vi "Fetch(Y)Trace.vi"(8 "error in (no error)":errorcluster, 11 "Keysight44xx in":refnum<class "Keysight44xx.lvclass">) -> (0 "error out":errorcluster, 2 "Waveform(s)":T1, 3 "Keysight44xx out":refnum<class "Keysight44xx.lvclass">)   [LabVIEW 2018, in "SpecAnPlugins.lvlib" / "Keysight44xx.lvclass"]
doc: "This function returns the trace the spectrum analyzer acquires. The trace is from a previously initiated acquisition. The user calls the Initiate function to start an acquisition. The user calls the Acquisition Status function to determine when the acquisition is complete. \n\nThe user may call the Read Y Trace function instead of the Initiate function. This function starts an acquisition, waits for the acquisition to complete, and returns the trace in one function call. \n\nThe Amplitude array returns data that represents the amplitude of the signals obtained by sweeping from the start frequency to the stop frequency (in frequency domain, in the time domain the amplitude array is ordered from beginning of sweep to end). The Amplitude Units attribute determines the units of the points in the Amplitude array.\n\nThis function does not check the instrument status. The user calls the Error Query function at the conclusion of the sequence to check the instrument status."
uses:
  Keysight44xx.lvclass
  C:/Users/ico/Documents/Projects/NistPluggableModules/SpecAn/SpecAnPlugins/SpecAnBaseClass/SpecAnBase.lvclass
  SpecAnBaseClass/Typedefs/Waveform(s).ctl
  SpecAnBaseClass/SpecAnBase.lvclass
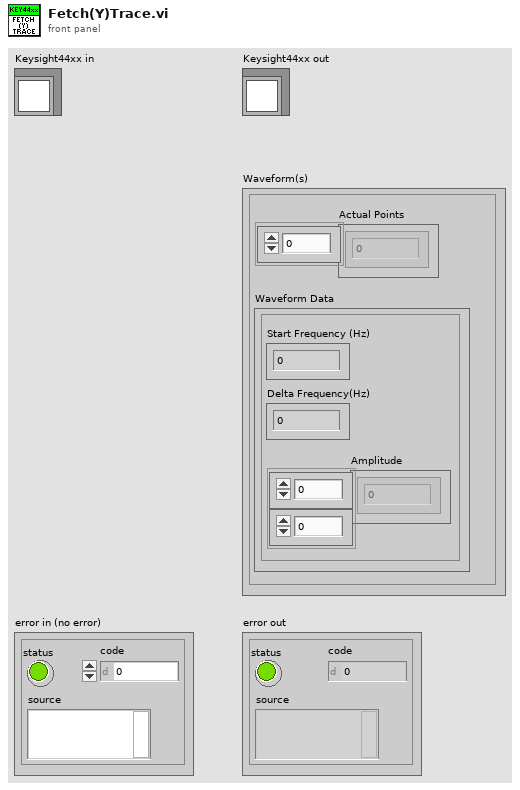
[diagram p1: front panel]
types:
  T1 = typedef "SpecAnPlugins.lvlib/SpecAnBase.lvclass/Waveform(s).ctl" = cluster{"Actual Points":i32[], "Waveform Data":cluster{"Start Frequency (Hz)":dbl, "Delta Frequency(Hz)":dbl, "Amplitude":dbl[][]}}
  T2 = typedef "SpecAnPlugins.lvlib/SpecAnBase.lvclass/Acquisition.ctl" = cluster{"Handle":string, "Connected":bool, "Enabled":bool, "SweepModeContinuous":bool, "NumberOfSweeps":i32, "DetectorTypeAuto":bool, "DetectorType":i32, "VerticalScale":i32, "MaximumTime(seconds)":dbl}
  T3 = typedef "SpecAnPlugins.lvlib/SpecAnBase.lvclass/Trace.ctl" = cluster{"TraceName":string, "TraceSize":i32, "TraceType":i32}[]
  T4 = typedef "SpecAnPlugins.lvlib/SpecAnBase.lvclass/Frequency.ctl" = cluster{"FrequencyStart":dbl, "FrequencyStop":dbl, "FrequencyOffset":dbl}
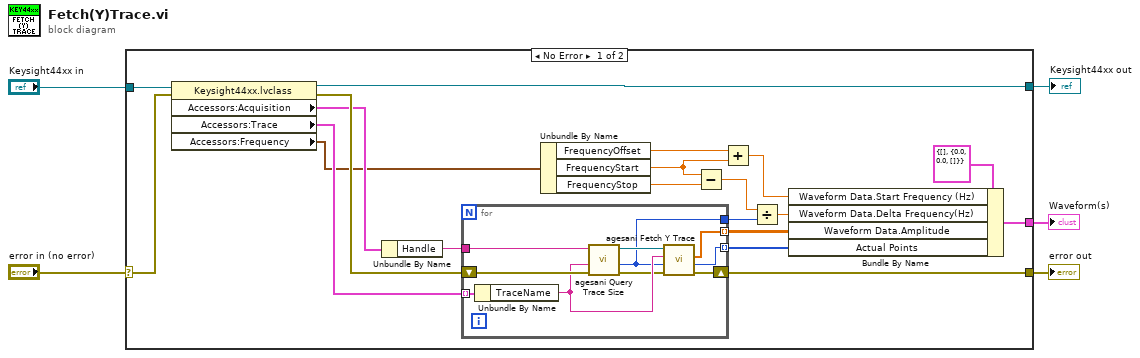
[diagram p0: block diagram]
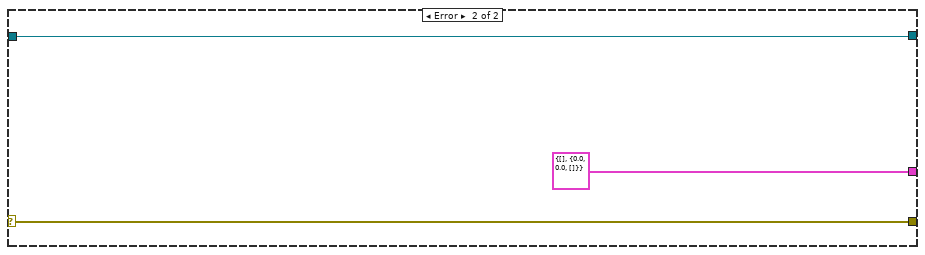
[diagram p2: hidden frame]
diagram:
  n1 = case shown="No Error" "error in (no error)" {
    selector: "error in (no error)" -> [w24 w38]
    tunnel: [w22 w38] -> w4
    tunnel: "Keysight44xx in" -> [w25 w37]
    tunnel: [w23 w37] -> w2
    tunnel: [w16 T1 {"Actual Points"=[], "Waveform Data"={"Start Frequency (Hz)"=0.0, "Delta Frequency(Hz)"=0.0, "Amplitude"=[]}} ("Waveform(s)")] -> w1
    frame No Error {
      n2 = property class="Keysight44xx.lvclass"(reference=w25, error in=w24) -> (reference out=w23:refnum<class "Keysight44xx.lvclass">, error out=w21:errorcluster, "Accessors:Acquisition"=w20:T2, "Accessors:Trace"=w18:T3, "Accessors:Frequency"=w13:T4)
      n3 = Unbundle By Name(w20) -> ("Handle"=w19:string)
      n4 = for {
        tunnel: w19 -> [w31]
        shift-right: [w35] -> w22
        shift-left: w21 -> [w33]
        tunnel: w18 -> [w34] mode=indexing
        tunnel: [w28] -> w15 mode=indexing
        tunnel: [w27] -> w14 mode=indexing
        tunnel: [w26] -> w10
        n5 = Unbundle By Name(w34) -> ("TraceName"=w32:string)
        n6 = call <instrlib>:"agesani Query Trace Size.vi"("error in (no error)"=w33, "trace name (\"\")"=w32, "instrument handle"=w31) -> ("error out"=w30:errorcluster, "trace size"=w26:i32, "instrument handle out"=w29:refnum<k15>)  [unwired: 6 out]
        n7 = call <instrlib>:"agesani Fetch Y Trace.vi"("error in (no error)"=w30, "array length"=w26, "trace name"=w32, "instrument handle"=w29) -> ("error out"=w35:errorcluster, "actual points"=w28:i32, "amplitude"=w27:dbl[])  [unwired: 4 in, 1 out]
      }
      n8 = Unbundle By Name(w13) -> ("FrequencyOffset"=w8:dbl, "FrequencyStart"=w7:dbl, "FrequencyStop"=w12:dbl)
      n9 = Subtract(x=w7, y=w12) -> (x-y=w11:dbl)
      n10 = Add(x=w8, y=w7) -> (x+y=w6:dbl)
      n11 = Divide(x=w11, y=w10) -> (x/y=w9:dbl)
      n12 = Bundle By Name(cluster=T1 {"Actual Points"=[], "Waveform Data"={"Start Frequency (Hz)"=0.0, "Delta Frequency(Hz)"=0.0, "Amplitude"=[]}} ("Waveform(s)"), "Waveform Data.Start Frequency (Hz)"=w6, "Waveform Data.Delta Frequency(Hz)"=w9, "Waveform Data.Amplitude"=w14, "Actual Points"=w15) -> (w16:T1)
    }
    frame Error {
    }
  }
  "error out" <- w4
  "Keysight44xx out" <- w2
  "Waveform(s)" <- w1
